vi "Read Grant Flow.vi"(8 "error in (no error)":errorcluster, 11 "Oauth2 in":refnum<class "Oauth2.lvclass">) -> (0 "error out":errorcluster, 2 "Grant Flow":T1, 3 "Oauth2 out":refnum<class "Oauth2.lvclass">)   [LabVIEW 2013, in "Oauth2.lvclass"]
uses:
  Oauth2.lvclass
  OAuth2 Flow -- enum.ctl
  OAuthToken/OAuth2 Token Element -- enum.ctl
  OAuthToken/OAuthAccessToken.lvclass
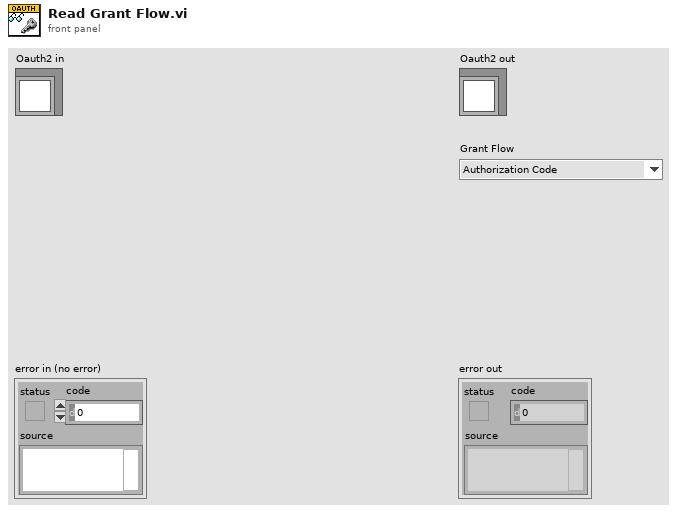
[diagram p1: front panel]
types:
  T1 = typedef "Oauth2.lvclass/OAuth2 Flow -- enum.ctl" = enum16{"Authorization Code", "Authorization Code (PKCE)", "Implicit", "Resource Owner Credentials", "Client Credentials"}
  T2 = typedef "OAuthAccessToken.lvclass/OAuth2 Token Element -- enum.ctl" = enum16{"client_id", "client_secret", "response_type", "scope", "redirect_uri", "error", "error_description", "error_uri", "grant_type", "code", "access_token", "token_type", "expires_in", "username", "password", "refresh_token", "endpoint element"}
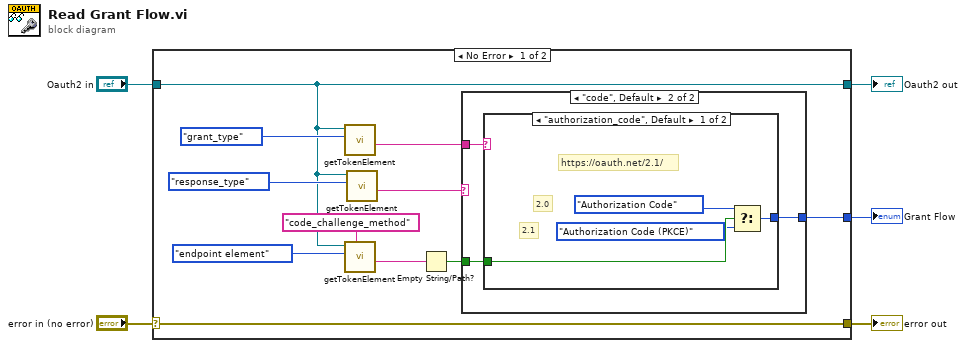
[diagram p0: block diagram]
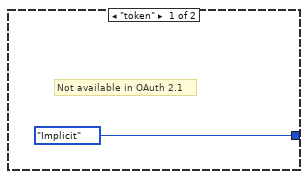
[diagram p2: hidden frame]
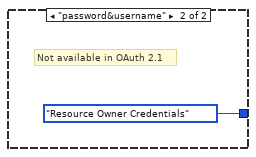
[diagram p3: hidden frame]
diagram:
  n1 = case shown="No Error" "error in (no error)" {
    selector: "error in (no error)" -> [w16 w26]
    tunnel: [w16 w26] -> w4
    tunnel: [w6 w27] -> w2
    tunnel: "Oauth2 in" -> [w6 w27]
    tunnel: [w10 _] -> w1
    frame No Error {
      n2 = call "getTokenElement.vi"("Token element"=OAuth2_Token_Element_--_enum."grant_type", "Oauth2 in"=w6) -> ("Value"=w9:string)  [unwired: 6 in, 3 out]
      n3 = call "getTokenElement.vi"("Endpoint Element Name"="code_challenge_method" ("argument"), "Token element"=OAuth2_Token_Element_--_enum."endpoint element", "Oauth2 in"=w6) -> ("Value"=w12:string)  [unwired: 5 in, 3 out]
      n4 = call "getTokenElement.vi"("Token element"=OAuth2_Token_Element_--_enum."response_type", "Oauth2 in"=w6) -> ("Value"=w7:string)  [unwired: 6 in, 3 out]
      n5 = Empty String/Path?(string/path=w12) -> (empty?=w11:bool)
      n6 = case shown="\"code\", Default" w7 {
        tunnel: w11 -> [_ w20]
        tunnel: [OAuth2_Flow_--_enum."Implicit" ("Grant Flow") w19] -> w10
        tunnel: w9 -> [_ w18]
        frame "token" {
          # "Not available in OAuth 2.1"
        }
        frame "code", Default {
          n7 = case shown="\"authorization_code\", Default" w18 {
            tunnel: w20 -> [w24 _]
            tunnel: [w21 OAuth2_Flow_--_enum."Resource Owner Credentials" ("Grant Flow")] -> w19
            frame "authorization_code", Default {
              # "https://oauth.net/2.1/"
              # "2.1"
              # "2.0"
              n8 = Select(t=OAuth2_Flow_--_enum."Authorization Code" ("Grant Flow"), s=w24, f=OAuth2_Flow_--_enum."Authorization Code (PKCE)" ("Grant Flow")) -> (s? t:f=w21:T1)
            }
            frame "password&username" {
              # "Not available in OAuth 2.1"
            }
          }
        }
      }
    }
    frame Error {
    }
  }
  "error out" <- w4
  "Oauth2 out" <- w2
  "Grant Flow" <- w1
